vi "PicoScope2000StartStreaming.vi"(7 "Acquisition Settings":T1 {"Time Units" items=["Nanoseconds (ns)", "Microseconds (us)", "Milliseconds (ms)", "Seconds (s)"]}, 8 "handle in":i16, 9 "error in":errorcluster) -> (0 "time_units":u32, 1 "Sample Interval":u32, 2 "handle out":i16, 3 "error out":errorcluster, 4 "Channel B":i16[](array[numeric]), 5 "Channel A":i16[](array[numeric]))   [LabVIEW 2009]
doc: "This VI starts the oscilloscope streaming. It outputs arrays that will contain samples once PicoScope3000aGetStreamingValues.vi has returned."
uses:
  ps2000Wrap.dll
  ps2000.dll
panel:
  # "Overview Buffer Size is the size of the temporary buffers used to\nstore data before returning it to the application."
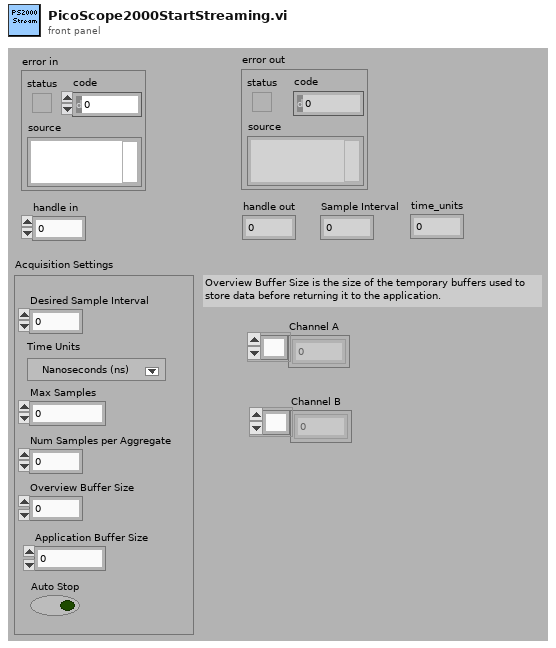
[diagram p1: front panel]
types:
  T1 = cluster{"Auto Stop":bool, "Desired Sample Interval":u32, "Max Samples":u32, "Num Samples per Aggregate":u32, "Overview Buffer Size":u32, "Time Units":u32, "Application Buffer Size":u32}
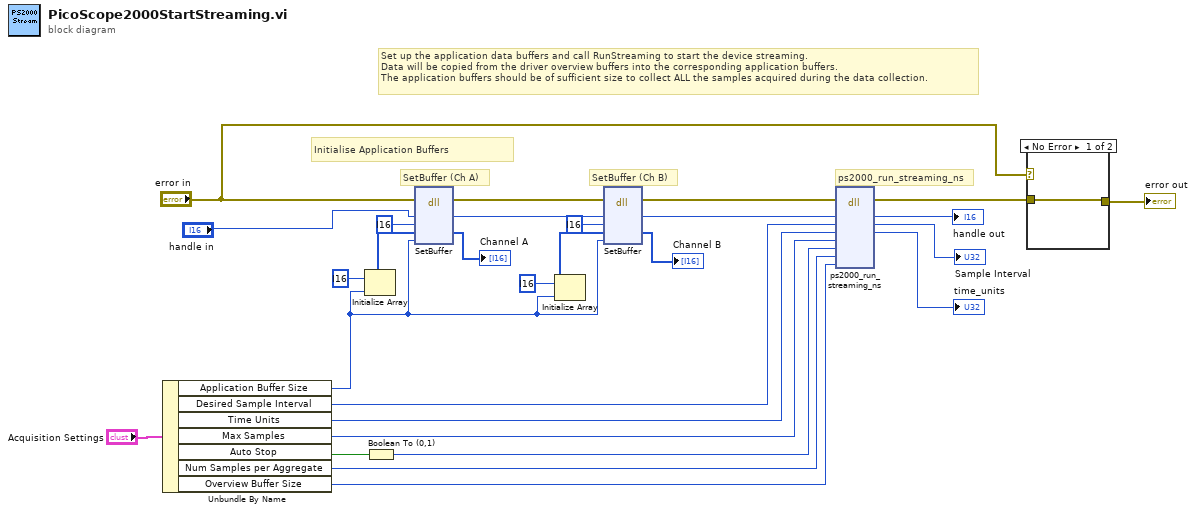
[diagram p0: block diagram]
diagram:
  # "ps2000_run_streaming_ns"
  # "SetBuffer (Ch B)"
  # "SetBuffer (Ch A)"
  # "Initialise Application Buffers"
  # "Set up the application data buffers and call RunStreaming to start the device streaming.\nData will be copied from the driver overview buffers into the corresponding application buffers.\nThe application buffers should be of sufficient size to collect ALL the samples acquired during the data collection."
  n1 = Unbundle By Name("Acquisition Settings") -> ("Application Buffer Size"=w4:u32, "Desired Sample Interval"=w10:u32, "Time Units"=w9:u32, "Max Samples"=w5:u32, "Auto Stop"=w27:bool, "Num Samples per Aggregate"=w7:u32, "Overview Buffer Size"=w6:u32)
  n2 = Initialize Array(i16 ? ("element"), w4) -> (w23:i16[])
  n3 = Boolean To (0,1)(Boolean=w27) -> (0, 1=w8:i16)
  n4 = dll-call lib="ps2000Wrap.dll" fn="SetBuffer" ("PS2000.dll:_ps2000_stop@4")(error in="error in", "handle"="handle in", "channel"=i16 ?, "buffer"=w23, "bufferSize"=w4) -> (error out=w17:errorcluster, "handle"=w21:i16, "buffer"=→"Channel A":i16[])  [unwired: 5 in, 1 out]
  n5 = Initialize Array(i16 ? ("element"), w4) -> (w19:i16[])
  n6 = dll-call lib="ps2000Wrap.dll" fn="SetBuffer" ("PS2000.dll:_ps2000_stop@4")(error in=w17, "handle"=w21, "channel"=i16 ?, "buffer"=w19, "bufferSize"=w4) -> (error out=w15:errorcluster, "handle"=w11:i16, "buffer"=→"Channel B":i16[])  [unwired: 5 in, 1 out]
  n7 = dll-call lib="PS2000.dll" fn="ps2000_run_streaming_ns"(error in=w15, "handle"=w11, "sample_interval"=w10, "time_units"=w9, "max_samples"=w5, "auto_stop"=w8, "noOfSamplesPerAggregate"=w7, "overview_buffer_size"=w6) -> (error out=w14:errorcluster, "handle"=→"handle out":i16, "sample_interval"=→"Sample Interval":u32, "time_units"=→"time_units":u32)  [unwired: 7 in, 1 out]
  n8 = case shown="No Error" "error in" {
    tunnel: [w29 w30] -> w28
    tunnel: w14 -> [w29 w30]
    frame #0 {
    }
    frame #1 {
    }
  }
  "error out" <- w28
